vi "Read Pulse Configuration.vi"(8 "error in (no error)":errorcluster, 11 "NI-Scope Lock-in Driver in":refnum<class "NI-Scope Lock-in Driver.lvclass">) -> (0 "error out":errorcluster, 2 "Configuration":T1={"Pre-trigger duration"=0.01, "Post-trigger duration"=0.1, "Rate"=1000000.0, "Ranges"=[10.0], "Re-name channels"=[], "Active channels"="0:1", "External clock"=FALSE} {"Rate" format="%#_8pHz"; "Post-trigger duration" format="%#_6ps"; "Pre-trigger duration" format="%#_6ps"; "Ranges" format="%#_6pV"}, 3 "NI-Scope Lock-in Driver out":refnum<class "NI-Scope Lock-in Driver.lvclass">)   [LabVIEW 2016, in "NI-Scope Lock-in Driver.lvclass"]
uses:
  NI-Scope Lock-in Driver.lvclass
  C:/github/NHMFL_Core/Libraries/Instruments/Instrument Driver/Instrument Driver.lvclass
  Instruments/Pulse Driver/Pusle Driver Configuration.ctl
  Instruments/Instrument Driver/Instrument Driver.lvclass/Instrument Driver.ctl
  Instruments/Instrument Driver/Read Cycle period.vi
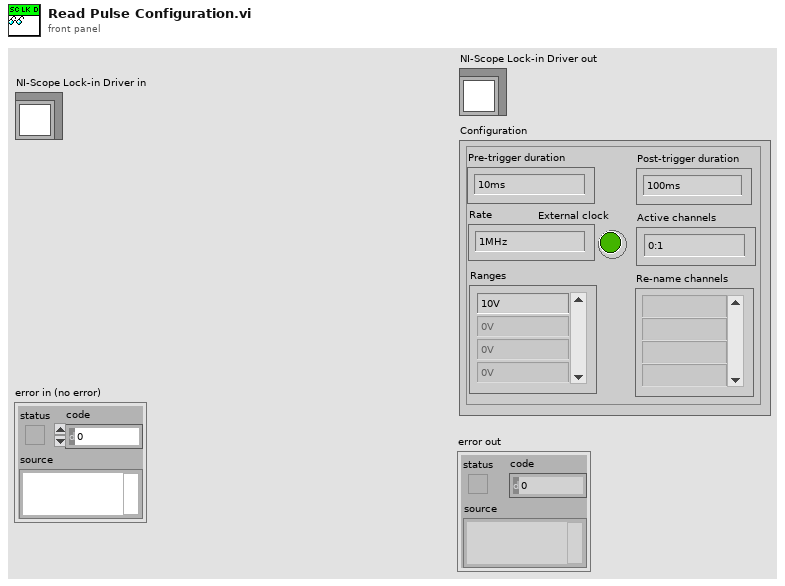
[diagram p1: front panel]
types:
  T1 = typedef "Pusle Driver Configuration.ctl" = cluster{"Pre-trigger duration":dbl, "Post-trigger duration":dbl, "Rate":dbl, "Ranges":dbl[], "Re-name channels":string[], "Active channels":string, "External clock":bool}
  T2 = typedef "NI-Scope Lock-in Configuration.ctl" = cluster{"Points per sine wave":i32, "Rate":dbl, "Re-name channels":string[], "Active channels":string, "Ranges":dbl[], "Sync on trigger":bool, "R-Q":bool}
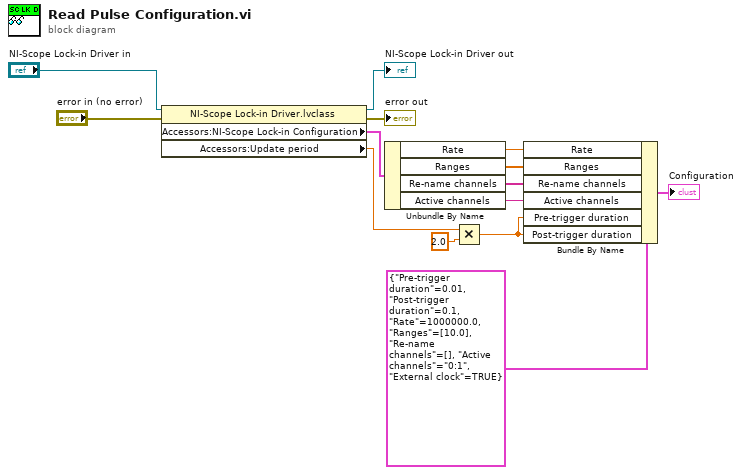
[diagram p0: block diagram]
diagram:
  n1 = property class="NI-Scope Lock-in Driver.lvclass"(reference="NI-Scope Lock-in Driver in", error in="error in (no error)") -> (reference out=→"NI-Scope Lock-in Driver out":refnum<class "NI-Scope Lock-in Driver.lvclass">, error out=→"error out":errorcluster, "Accessors:NI-Scope Lock-in Configuration"=w2:T2, "Accessors:Update period"=w9:dbl)
  n2 = Unbundle By Name(w2) -> ("Rate"=w7:dbl, "Ranges"=w6:dbl[], "Re-name channels"=w5:string[], "Active channels"=w4:string)
  n3 = Multiply(x=w9, y=2.0) -> (x*y=w1:dbl)
  n4 = Bundle By Name(cluster=T1 {"Pre-trigger duration"=0.01, "Post-trigger duration"=0.1, "Rate"=1000000.0, "Ranges"=[10.0], "Re-name channels"=[], "Active channels"="0:1", "External clock"=TRUE} ("Pulse Configuration"), "Rate"=w7, "Ranges"=w6, "Re-name channels"=w5, "Active channels"=w4, "Pre-trigger duration"=w1, "Post-trigger duration"=w1) -> (→"Configuration":T1)
